vi "Create.vi"(9 "jettl":refnum<class "jettl.lvclass">, 10 "Self Alias":string) -> (2 "Msg Strategy":refnum<class "Msg Strategy.lvclass">)   [LabVIEW 2021, in "Create Msg Strategy.lvlib"]
uses:
  Create Msg Strategy.lvlib
  Create Msg Strategy/Create Msg Strategy.lvclass
  C:/git/jettl/jettl/Create Msg Strategy/Create Msg Strategy/Create Msg Strategy.lvclass
  C:/git/jettl/jettl/jettl/Msg Strategy/Msg Strategy.lvclass
  jettl/Msg Strategy/Msg Strategy.lvclass
  jettl/jettl/jettl.lvclass
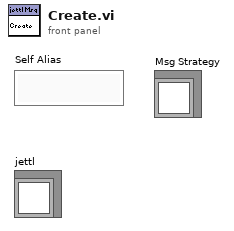
[diagram p1: front panel]
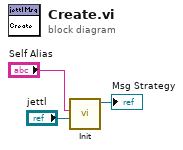
[diagram p0: block diagram]
diagram:
  n1 = call "Init.vi"("jettl"="jettl", "Self Alias"="Self Alias") -> ("Create Msg Strategy out"=→"Msg Strategy":refnum<class "Create Msg Strategy.lvclass">)  [unwired: 9 in]
